vi "Fire Alarm System - 2 Ifs Serial.vi"() -> ()   [LabVIEW 2021]
uses:
  <vilib>/MakerHub/LINX/Public/Peripherals/Analog/Analog Read 1 Chan.vi
  <vilib>/MakerHub/LINX/Public/Peripherals/Digital/Digital Write 1 Chan.vi
  <vilib>/MakerHub/LINX/Public/Peripherals/Digital/Digital Read 1 Chan.vi
  <vilib>/MakerHub/LINX/Public/Peripherals/PWM/PWM Set Duty Cycle 1 Chan.vi
  <vilib>/MakerHub/LINX/Public/Peripherals/Digital/Digital Write N Chans.vi
  <vilib>/MakerHub/LINX/Public/Peripherals/Analog/Analog Read N Chans.vi
  <vilib>/MakerHub/LINX/Public/Peripherals/Digital/Digital Read N Chans.vi
  <vilib>/MakerHub/LINX/Private/Local IO/LinxDigitalWrite.vi
  <vilib>/MakerHub/LINX/Public/Utilities/Check Channel.vi
  <vilib>/MakerHub/LINX/Private/Local IO/LinxAnalogRead.vi
  <vilib>/MakerHub/LINX/Private/Local IO/LinxDigitalRead.vi
  <vilib>/MakerHub/LINX/Public/Utilities/Open Serial.vi
  <vilib>/MakerHub/LINX/Private/Utilties/Generate Error.vi
  <vilib>/MakerHub/LINX/Public/Sensors/Temperature/TMP3x/TMP35.vi
  <vilib>/MakerHub/LINX/Public/Peripherals/PWM/PWM Set Duty Cycle N Chans.vi
  <vilib>/MakerHub/LINX/LMH-LINX.lvlib
  <vilib>/MakerHub/LINX/Public/Sensors/Temperature/TMP3x/TMP3x.lvlib
panel:
  out "Boolean":bool
  in  "Buzzer":u8
  in  "Pump":dbl(knob) scale=0.0..1.0
  in  "Motor Direction 2":bool[](array[boolean]) caption="Motor Direction"
  in  "PWM Channel 2":u8
  out "Error Out":errorcluster
  in  "Motor Speed":dbl(knob) scale=0.0..1.0
  in  "Motor Direction":bool[](array[boolean])
  in  "PWM Channel":u8
  out "Waveform Chart":dbl(graph)
  out "Meter":dbl(knob) scale=0.0..10.0
  in  "Analog Channel 3":u8
  out "Fire":bool
  in  "DO Channel 2":u8
  in  "DI Channel":u8
  out "Thermometer":u8(slide) scale=0.0..100.0
  in  "Temperature A. Channel":u8
  out "Temp C":dbl format="%#.1g"
  in  "stop":bool
  in  "Smoke LED DO Channel":u8
  out "Smoke":bool
  in  "Serial Port":refnum<visa-resource-name>="N/A"
  in  "Smoke Reference Value":dbl
  out "Smoke o/p":dbl
  in  "Analog Channel":u8
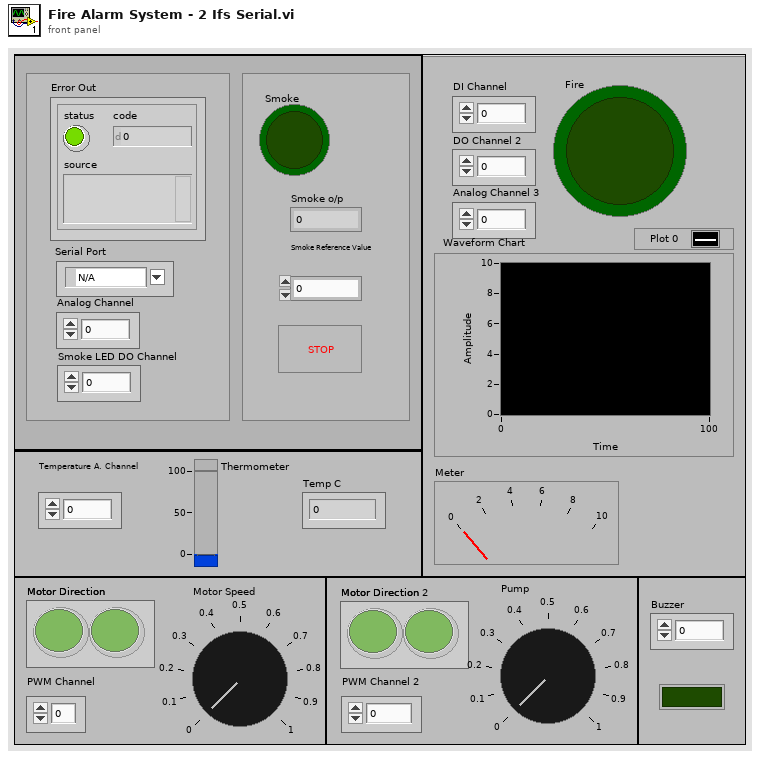
[diagram p1: front panel]
types:
  T1 = typedef "LMH-LINX.lvlib/LINX Ref.ctl" = cluster{"IO":T2, "Interface":T3, "LINX Device Config":T4}
  T2 = typedef "LMH-LINX.lvlib/Platform.ctl" = enum16{"Remote", "Local"}
  T3 = typedef "LMH-LINX.lvlib/Interface.ctl" = enum16{"Serial", "TCP"}
  T4 = typedef "LMH-LINX.lvlib/Device.lvlib/LINX Device Config.ctl" = cluster{"Interface":T3, "COM Port":refnum<visa-resource-name>, "TCP Configuration":T5, "Device Family":u8, "Device ID":u8, "Device Name":string, "TCP Ref":refnum<k5>, "Channels":T6}
  T5 = typedef "LMH-LINX.lvlib/Device.lvlib/TCP Config.ctl" = cluster{"IP Address":string, "Port":u16}
  T6 = typedef "LMH-LINX.lvlib/Channels.ctl" = cluster{"DI":u8[], "DO":u8[], "AI":u8[], "AO":u8[], "PWM":u8[], "QE":u8[], "UART":u8[], "I2C 2":u8[], "SPI":u8[], "CAN":u8[], "Servo":u8[], "AI Ref (V)":dbl, "AI Resolution (Bits)":u8, "AO Ref (V)":dbl, "AO Resolution (Bits)":u8}
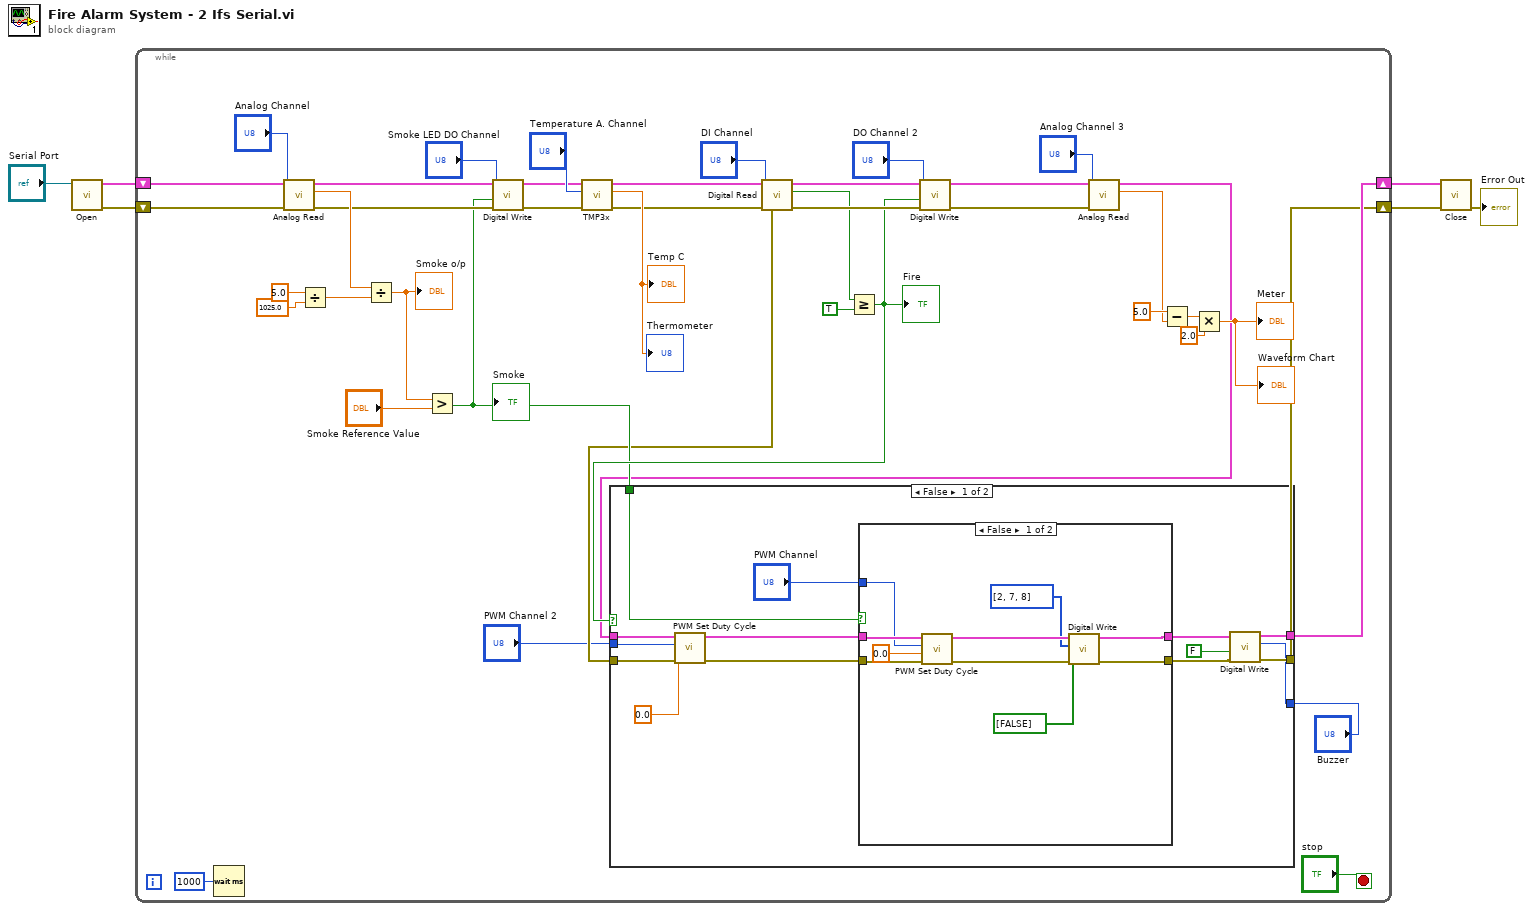
[diagram p0: block diagram]
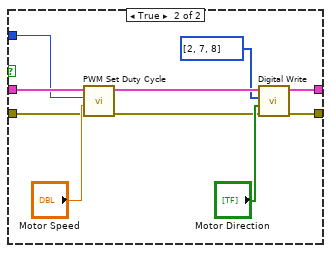
[diagram p2: hidden frame]
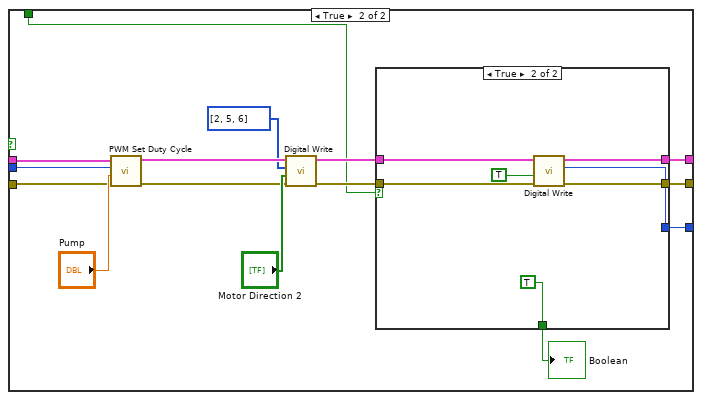
[diagram p3: hidden frame]
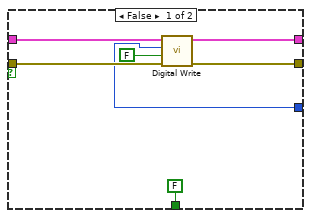
[diagram p4: hidden frame]
diagram:
  n1 = call-poly <vilib>:"Open.vi"("Serial Port"="Serial Port") -> ("Error Out"=w5:errorcluster, "LINX Resource"=w4:T1)  [unwired: 8 in, 1 out]
  n2 = while {
    shift-right: [w9] -> w2
    shift-left: w5 -> [w13]
    shift-right: [w10] -> w3
    shift-left: w4 -> [w14]
    stop <- "stop" stop-if-true
    n3 = Wait (ms)(milliseconds to wait=u32 1000) -> ()  [unwired: 1 out]
    n4 = call-poly <vilib>:"Analog Read.vi"("Error In"=w13, "Analog Channel"="Analog Channel", "LINX Resource"=w14) -> ("Error Out"=w41:errorcluster, "Voltage"=w46:dbl, "LINX Resource"=w42:T1)  [unwired: 5 in, 1 out]
    n5 = Divide(x=5.0, y=1025.0) -> (x/y=w47:dbl)
    n6 = Divide(x=w46, y=w47) -> (x/y=w37:dbl)
    "Smoke o/p" <- w37
    n7 = Greater?(x=w37, y="Smoke Reference Value") -> (0:w15:bool)
    "Smoke" <- w15
    n8 = call-poly <vilib>:"Digital Write.vi"("Error In"=w41, "Output Value"=w15, "DO Channel"="Smoke LED DO Channel", "LINX Resource"=w42) -> ("Error Out"=w34:errorcluster, "LINX Resource"=w35:T1)  [unwired: 6 in]
    n9 = call-poly <vilib>:"TMP3x.vi"("Error In"=w34, "Analog Channel"="Temperature A. Channel", "LINX Resource"=w35) -> ("Error Out"=w20:errorcluster, "Temp C"=→"Temp C" →"Thermometer":dbl, "LINX Resource"=w21:T1)  [unwired: 6 in]
    n10 = call-poly <vilib>:"Digital Read.vi"("Error In"=w20, "DI Channel"="DI Channel", "LINX Resource"=w21) -> ("Error Out"=w31:errorcluster, "DI Value"=w23:bool, "LINX Resource"=w32:T1)  [unwired: 6 in]
    n11 = Greater Or Equal?(x=w23, y=TRUE) -> (x >= y?=w16:bool)
    "Fire" <- w16
    n12 = call-poly <vilib>:"Digital Write.vi"("Error In"=w31, "Output Value"=w16, "DO Channel"="DO Channel 2", "LINX Resource"=w32) -> ("Error Out"=w27:errorcluster, "LINX Resource"=w28:T1)  [unwired: 6 in]
    n13 = call-poly <vilib>:"Analog Read.vi"("Error In"=w27, "Analog Channel"="Analog Channel 3", "LINX Resource"=w28) -> ("Error Out"=w11:errorcluster, "Voltage"=w24:dbl, "LINX Resource"=w12:T1)  [unwired: 5 in, 1 out]
    n14 = case shown="False" w16 {
      tunnel: w15 -> [w62 w86]
      tunnel: w12 -> [w61 w92]
      tunnel: w11 -> [w60 w91]
      tunnel: [w51 w87] -> w9
      tunnel: [w50 w88] -> w10
      tunnel: "PWM Channel 2" -> [w56 w84]
      tunnel: "Buzzer" -> [w49 w83]
      frame False {
        n15 = call-poly <vilib>:"PWM Set Duty Cycle.vi"("Error In"=w60, "Duty Cycle (0-1)"=0.0, "PWM Channel"=w56, "LINX Resource"=w61) -> ("Error Out"=w57:errorcluster, "LINX Resource"=w58:T1)  [unwired: 6 in]
        n16 = case shown="False" w62 {
          tunnel: [w64 w77] -> w53
          tunnel: [w63 w76] -> w52
          tunnel: w58 -> [w67 w75]
          tunnel: w57 -> [w66 w74]
          tunnel: "PWM Channel" -> [w65 w73]
          frame False {
            n17 = call-poly <vilib>:"PWM Set Duty Cycle.vi"("Error In"=w66, "Duty Cycle (0-1)"=0.0, "PWM Channel"=w65, "LINX Resource"=w67) -> ("Error Out"=w72:errorcluster, "LINX Resource"=w71:T1)  [unwired: 6 in]
            n18 = call-poly <vilib>:"Digital Write.vi"("Error In"=w72, "Values"=bool[] [FALSE], "DO Channels"=i32[] [2, 7, 8], "LINX Resource"=w71) -> ("Error Out"=w63:errorcluster, "LINX Resource"=w64:T1)  [unwired: 6 in]
          }
          frame True {
            n19 = call-poly <vilib>:"PWM Set Duty Cycle.vi"("Error In"=w74, "Duty Cycle (0-1)"="Motor Speed", "PWM Channel"=w73, "LINX Resource"=w75) -> ("Error Out"=w80:errorcluster, "LINX Resource"=w79:T1)  [unwired: 6 in]
            n20 = call-poly <vilib>:"Digital Write.vi"("Error In"=w80, "Values"="Motor Direction", "DO Channels"=i32[] [2, 7, 8], "LINX Resource"=w79) -> ("Error Out"=w76:errorcluster, "LINX Resource"=w77:T1)  [unwired: 6 in]
          }
        }
        n21 = call-poly <vilib>:"Digital Write.vi"("Error In"=w52, "Output Value"=FALSE, "DO Channel"=w49, "LINX Resource"=w53) -> ("Error Out"=w51:errorcluster, "LINX Resource"=w50:T1)  [unwired: 6 in]
      }
      frame True {
        n22 = call-poly <vilib>:"PWM Set Duty Cycle.vi"("Error In"=w91, "Duty Cycle (0-1)"="Pump", "PWM Channel"=w84, "LINX Resource"=w92) -> ("Error Out"=w95:errorcluster, "LINX Resource"=w94:T1)  [unwired: 6 in]
        n23 = call-poly <vilib>:"Digital Write.vi"("Error In"=w95, "Values"="Motor Direction 2", "DO Channels"=i32[] [2, 5, 6], "LINX Resource"=w94) -> ("Error Out"=w89:errorcluster, "LINX Resource"=w90:T1)  [unwired: 6 in]
        n24 = case shown="True" w86 {
          tunnel: w90 -> [w103 w109]
          tunnel: w89 -> [w100 w108]
          tunnel: [w102 w111] -> w88
          tunnel: [w101 w110] -> w87
          tunnel: [FALSE ("Boolean") TRUE ("Boolean")] -> w85
          tunnel: w83 -> [w98 w105]
          frame False {
            n25 = call-poly <vilib>:"Digital Write.vi"("Error In"=w100, "Output Value"=FALSE, "DO Channel"=w98, "LINX Resource"=w103) -> ("Error Out"=w101:errorcluster, "LINX Resource"=w102:T1)  [unwired: 6 in]
          }
          frame True {
            n26 = call-poly <vilib>:"Digital Write.vi"("Error In"=w108, "Output Value"=TRUE, "DO Channel"=w105, "LINX Resource"=w109) -> ("Error Out"=w110:errorcluster, "LINX Resource"=w111:T1)  [unwired: 6 in]
          }
        }
        "Boolean" <- w85
      }
    }
    n27 = Subtract(x=5.0, y=w24) -> (x-y=w19:dbl)
    n28 = Multiply(x=w19, y=2.0) -> (x*y=→"Meter" →"Waveform Chart":dbl)
  }
  n29 = call <vilib>:"Close.vi"("Error In"=w2, "LINX Resource"=w3) -> ("Error Out"=→"Error Out":errorcluster)  [unwired: 9 in]
